vi "Get SMO Serial Number.vi"(8 "error in (no error)":errorcluster, 11 "Instrument in":refnum<class "Instrument.lvclass">) -> (0 "error out":errorcluster, 2 "Serial Number":string, 3 "Instrument out":refnum<class "Instrument.lvclass">)   [LabVIEW 2019, in "Instrument.lvclass"]
doc: "Override this VI to return the serial number of your Instrument"
uses:
  Instrument.lvclass
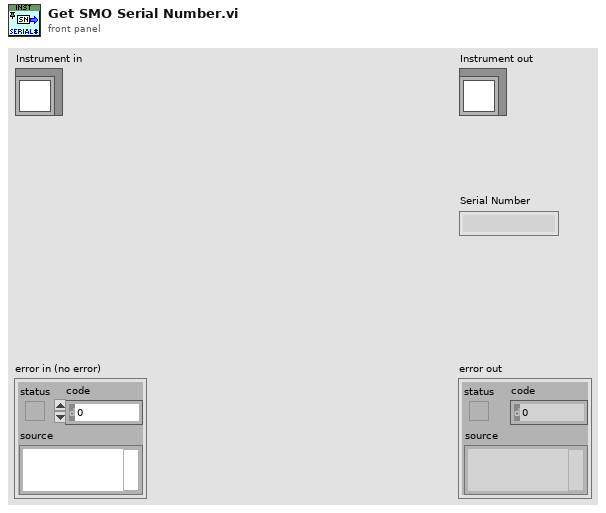
[diagram p1: front panel]
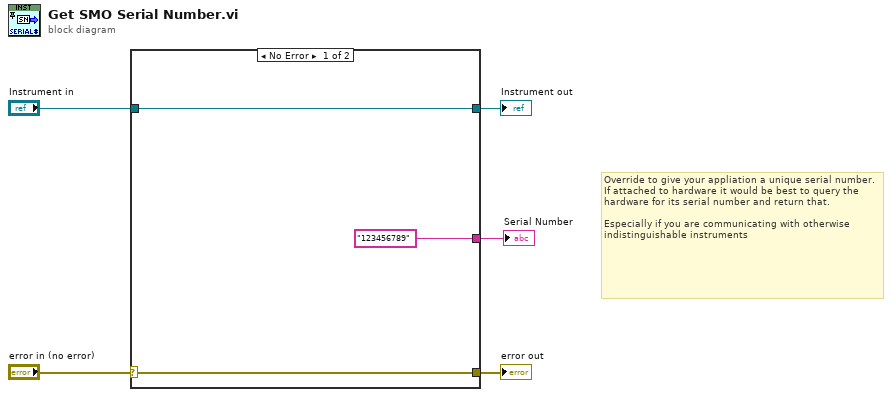
[diagram p0: block diagram]
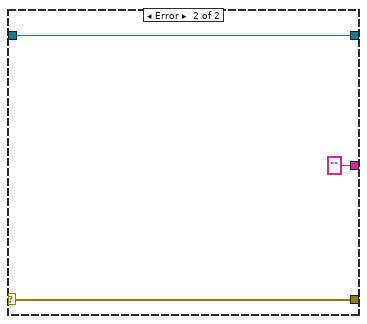
[diagram p2: hidden frame]
diagram:
  # "Override to give your appliation a unique serial number.\nIf attached to hardware it would be best to query the\nhardware for its serial number and return that. \n\nEspecially if you are communicating with otherwise \nindistinguishable instruments"
  n1 = case shown="No Error" "error in (no error)" {
    selector: "error in (no error)" -> [w8 w11]
    tunnel: [w8 w11] -> w4
    tunnel: [w7 w10] -> w2
    tunnel: "Instrument in" -> [w7 w10]
    tunnel: ["123456789" ("Serial Number") "" ("Serial Number")] -> w1
    frame No Error {
    }
    frame Error {
    }
  }
  "error out" <- w4
  "Instrument out" <- w2
  "Serial Number" <- w1
